vi "StepsList.vi"(0 "session in":refnum<k35>, 5 "Ticket Name":string, 11 "error in":errorcluster) -> (4 "session out":refnum<k35>, 8 "return value":T1(array[cluster]), 15 "error out":errorcluster)   [LabVIEW 2023]
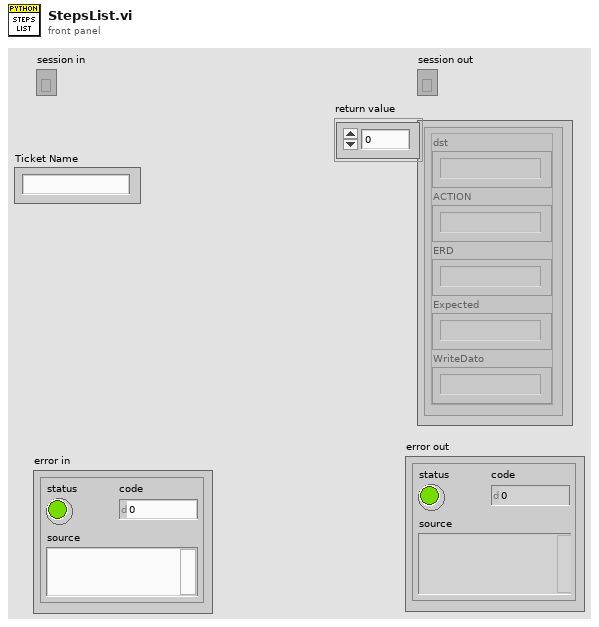
[diagram p1: front panel]
types:
  T1 = cluster{"dst":string, "ACTION":string, "ERD":string, "Expected":string, "WriteDato":string}[]
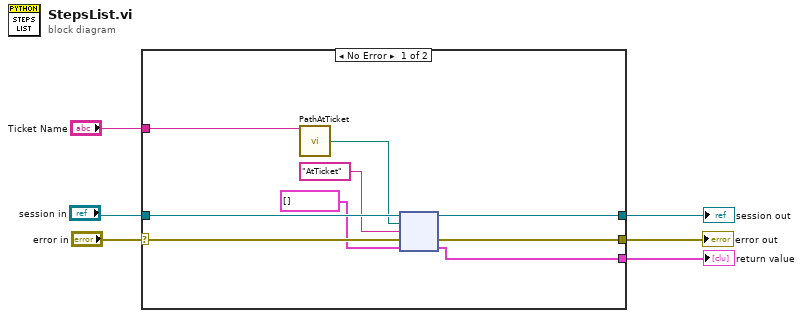
[diagram p0: block diagram]
diagram:
  n1 = case shown="No Error" "error in" {
    selector: "error in" -> [w15 w17]
    tunnel: [w13 w17] -> w6
    tunnel: "session in" -> [w14 w16]
    tunnel: [w12 w16] -> w3
    tunnel: [w9 _] -> w2
    tunnel: "Ticket Name" -> [w7 _]
    frame No Error {
      n2 = call "PathAtTicket.vi"("Ticket Name"=w7) -> ("path"=w8:path)  [unwired: 14 in]
      n3 = node(w14, w8, "AtTicket" ("function name"), w15, T1 []) -> (w12:refnum<k35>, w13:errorcluster, w9:T1)  [unwired: 2 out]
    }
    frame Error {
    }
  }
  "error out" <- w6
  "session out" <- w3
  "return value" <- w2
